vi "GetPointString.vi"(7 "Decoded String":string) -> (3 "Array":bool[][](array[boolean]))   [LabVIEW 2016]
panel:
  out "error out":errorcluster
  in  "error in (no error)":errorcluster
  out "new picture 2":picture
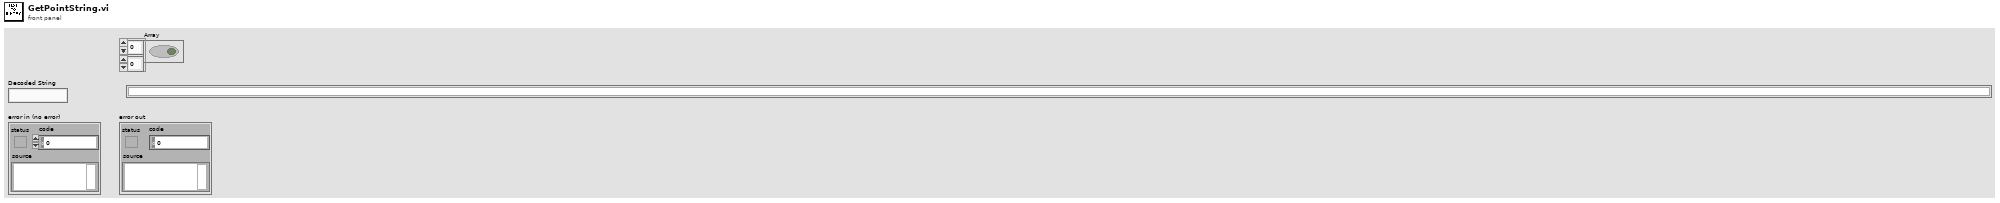
[diagram p1: front panel]
types:
  T1 = cluster{"Font Name:":string, "Size":i16, "Strikeout?":bool, "Italic?":bool, "Underline?":bool, "Outline?":bool, "Shadow?":bool, "Bold?":bool}
  T2 = enum16{"User-specified Font", "Application Font", "System Font", "Dialog Font"}
  T3 = cluster{"left":i16, "top":i16, "right":i16, "bottom":i16}
  T4 = typedef "imagedata.ctl" = cluster{"image type":i32, "image depth":i32, "image":u8[], "mask":u8[], "colors":u32[], "Rectangle":cluster{"left":i16, "top":i16, "right":i16, "bottom":i16}}
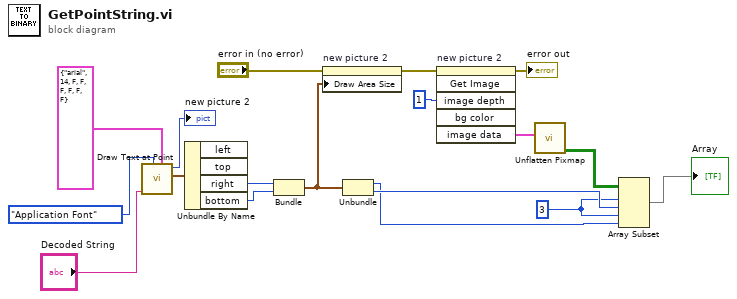
[diagram p0: block diagram]
diagram:
  w4 = 3 ("index")
  n1 = call <vilib>:"Draw Text at Point.vi"("[user-specified font]"=T1 {"Font Name:"="arial", "Size"=14, "Strikeout?"=FALSE, "Italic?"=FALSE, "Underline?"=FALSE, "Outline?"=FALSE, "Shadow?"=FALSE, "Bold?"=FALSE}, "desired font(Application)"=T2."Application Font", "text"="Decoded String") -> ("text rect"=w6:T3, "new picture"=→"new picture 2":picture)  [unwired: 6 in, 1 out]
  n2 = Unbundle By Name(w6) -> ("right"=w11:i16, "bottom"=w12:i16)  [unwired: 2 out]
  n3 = Bundle("right"=w11, "bottom"=w12) -> (w13:cluster{"right":i16, "bottom":i16})  [unwired: 1 in]
  n4 = property on="new picture 2" class="Pict"(error in="error in (no error)", "Draw Area Size"=w13) -> (error out=w16:errorcluster)  [unwired: 1 in, 1 out]
  n5 = Unbundle(w13) -> ("right"=w14:i16, "bottom"=w15:i16)
  n6 = invoke on="new picture 2" class="Pict" method="Get Image"(error in=w16, "image depth"=1 ("Image Depth")) -> (error out=→"error out":errorcluster, "image data"=w8:T4)  [unwired: 4 in, 4 out]
  n7 = call <vilib>:"Unflatten Pixmap.vi"("image data"=w8) -> ("1-bit pixmap"=w9:bool[][])  [unwired: 4 in, 6 out]
  n8 = Array Subset(array=w9, index (row)=w4, length (row)=w15, index (col)=w4, length (col)=w14) -> (→"Array":bool[][])
